vi "POP send QUIT.vi"(3 "error in":errorcluster, 5 "connection ID in":refnum<k5>) -> (0 "error out":errorcluster, 1 "QUIT response":string="\r\n", 2 "connection ID out":refnum<k5>)   [LabVIEW 2012]
doc: "This low-level POP VI sends the \"QUIT\" command to a mail server, terminating the TCP/IP connection. The connection can also be killed on the LabVIEW end through the use of the TCP Close Connection VI."
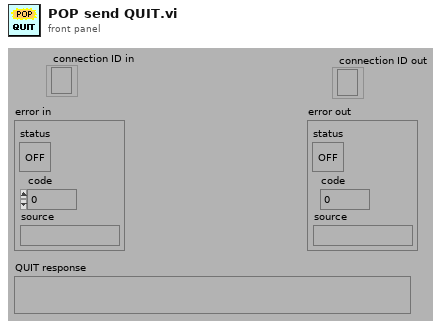
[diagram p1: front panel]
types:
  T1 = enum16{"Standard", "Buffered", "CRLF", "Immediate"}
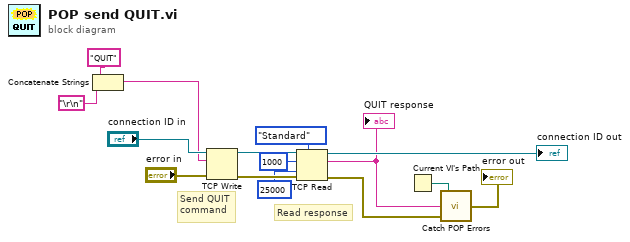
[diagram p0: block diagram]
diagram:
  # "Read response"
  # "Send QUIT\ncommand"
  n1 = Concatenate Strings("QUIT", "\r\n") -> (w7:string)
  n2 = TCP Write(connection ID="connection ID in", data in=w7, error in (no error)="error in") -> (connection ID out=w14:refnum<k5>, error out=w13:errorcluster)  [unwired: 1 in, 1 out]
  n3 = TCP Read(connection ID=w14, bytes to read=1000, error in (no error)=w13, 7:T1."Standard" ("mode (standard)"), 9:25000 ("timeout ms (25000)")) -> (connection ID out=→"connection ID out":refnum<k5>, data out=w3:string, error out=w2:errorcluster)
  "QUIT response" <- w3
  n4 = Current VI's Path() -> (path=w4:path)
  n5 = call "Catch POP Errors.vi"("error in"=w2, "POP server response"=w3, "Caller Path"=w4) -> ("error out"=→"error out":errorcluster)
